vi "GetJSONData.vi"(0 "reference in":refnum<class "Progressbar.lvclass">, 2 "VI Reference":refnum<vi>, 5 "error in (no error)":errorcluster) -> (14 "reference out":refnum<class "Progressbar.lvclass">, 15 "JSON string":string, 19 "error out":errorcluster)   [LabVIEW 2014, in "Progressbar.lvclass"]
uses:
  Progressbar.lvclass
  Object_class/Object.lvclass
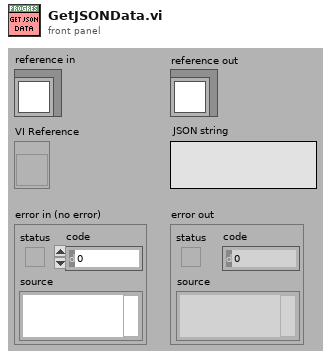
[diagram p1: front panel]
types:
  T1 = typedef "Object.lvclass/Attributes.ctl" = cluster{"UID":i32, "Type":string, "Coordinates":T2, "Reference":refnum<vi>}
  T2 = typedef "Object.lvclass/Coordinates.ctl" = cluster{"Left":i32, "Top":i32, "Height":u32, "Width":u32}
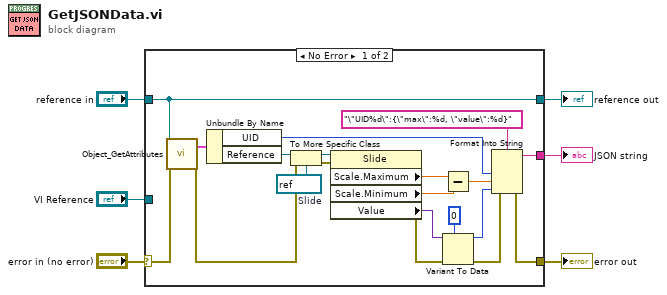
[diagram p0: block diagram]
diagram:
  n1 = case shown="No Error" "error in (no error)" {
    selector: "error in (no error)" -> [w24 w28]
    tunnel: [w25 w28] -> w5
    tunnel: [w16 w27] -> w3
    tunnel: "reference in" -> [w16 w27]
    tunnel: "VI Reference" -> [_ _]
    tunnel: [w17 _] -> w1
    frame No Error {
      w11 = refnum<vi> refnum  # Slide
      n2 = call "Object_GetAttributes.vi"("reference in"=w16, "error in (no error)"=w24) -> ("Data"=w15:T1, "error out"=w22:errorcluster)  [unwired: 14 in, 2 out]
      n3 = Unbundle By Name(w15) -> ("UID"=w14:i32, "Reference"=w13:refnum<vi>)
      n4 = To More Specific Class(target class=w11, reference=w13, error in=w22) -> (specific class reference=w12:refnum<vi>, error out=w23:errorcluster)
      n5 = property class="Slide"(reference=w12, error in=w23) -> (error out=w21:errorcluster, "Scale.Maximum"=w9:dbl, "Scale.Minimum"=w8:dbl, "Value"=w10:variant)  [unwired: 1 out]
      n6 = Subtract(x=w9, y=w8) -> (x-y=w7:dbl)
      n7 = Variant To Data(error in=w21, type=0, Variant=w10) -> (data=w18:i32, error out=w26:errorcluster)
      n8 = Format Into String(format string="\"UID%d\":{\"max\":%d, \"value\":%d}", error in=w26, w14, w7, w18) -> (resulting string=w17:string, error out=w25:errorcluster)  [unwired: 1 in]
    }
    frame Error {
    }
  }
  "error out" <- w5
  "reference out" <- w3
  "JSON string" <- w1
